vi "SPARK Configure Soft Limit.vi"   [LabVIEW 2023]
doc: "Configure a soft limit on the SPARK."
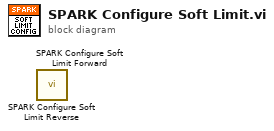
[diagram p0: block diagram]
diagram:
  n1 = call "SPARK Configure Soft Limit Reverse.vi"() -> ()  [unwired: 10 in, 2 out]
  n2 = call "SPARK Configure Soft Limit Forward.vi"() -> ()  [unwired: 10 in, 2 out]
